vi "Create.vi"(6 "exchange name":string, 7 "instance name":string, 8 "error in (no error)":errorcluster, 11 "service name":string) -> (0 "error out":errorcluster, 3 "publisher":refnum<class "IcmMessagePublisher.lvclass">)   [LabVIEW 2017, in "IcmMessagePublisher.lvclass"]
doc: "Creates an NI InsightCM Publisher message bus session."
uses:
  <vilib>/addons/InsightCM/MessageBus/MessagePublisher/IcmMessagePublisher.lvclass
  <vilib>/addons/InsightCM/MessageBus/MessagePublisher/controls/MessagePublisherData.ctl
  C:/Program Files (x86)/National Instruments/LabVIEW 2017/vi.lib/addons/InsightCM/Binaries/LabviewMessageAdapter.dll
  Binaries/LabviewMessageAdapter.dll
  <vilib>/addons/InsightCM/MessageBus/MessagePublisher/IcmMessagePublisher.lvclass/IcmMessagePublisher.ctl
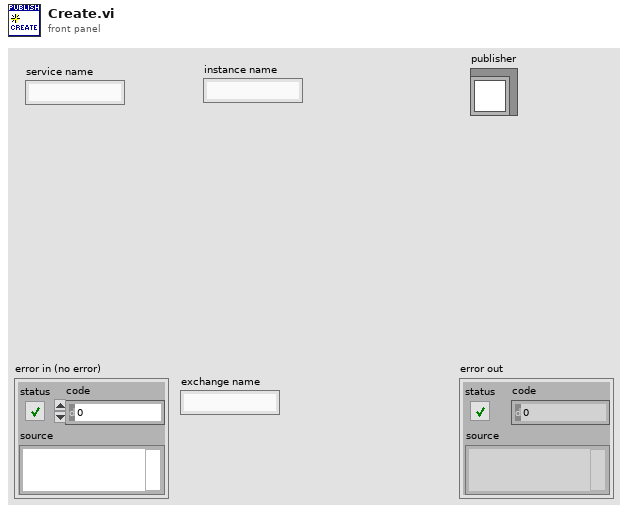
[diagram p1: front panel]
types:
  T1 = typedef "MessagePublisherData.ctl" = cluster{"Publisher":refnum<k24>}
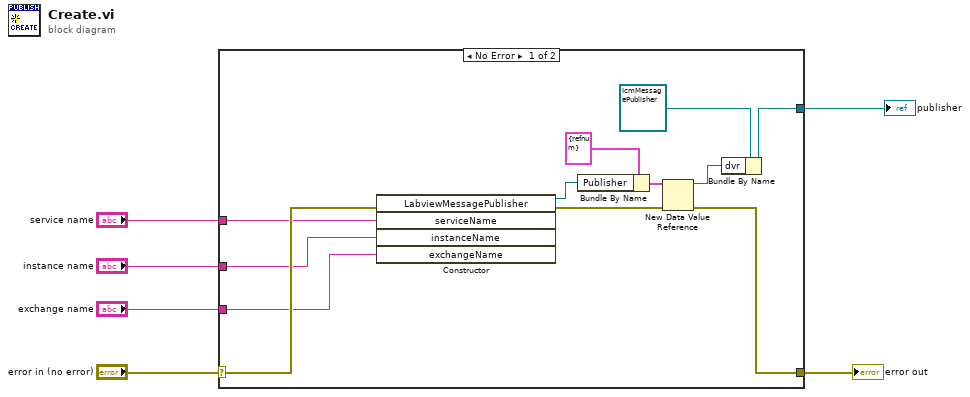
[diagram p0: block diagram]
diagram:
  n1 = case shown="No Error" "error in (no error)" {
    selector: "error in (no error)" -> [w11 w19]
    tunnel: [w10 w19] -> w5
    tunnel: [w12 _] -> w4
    tunnel: "service name" -> [w9 _]
    tunnel: "instance name" -> [w8 _]
    tunnel: "exchange name" -> [w7 _]
    frame No Error {
      n2 = constructor class="LabviewMessagePublisher"(error in=w11, "serviceName"=w9, "instanceName"=w8, "exchangeName"=w7) -> (reference out=w16:refnum<k24>, error out=w17:errorcluster)  [unwired: 2 in, 4 out]
      n3 = Bundle By Name(cluster=T1 {"Publisher"=refnum} ("Publisher"), "Publisher"=w16) -> (w18:T1)
      n4 = New Data Value Reference(data value=w18, error in=w17) -> (data value reference=w15:refnum<data-value>, error out=w10:errorcluster)
      n5 = Bundle By Name(cluster=refnum<class "IcmMessagePublisher.lvclass"> refnum ("IcmMessagePublisher in"), "dvr"=w15) -> (w12:refnum<class "IcmMessagePublisher.lvclass">)
    }
    frame Error {
    }
  }
  "error out" <- w5
  "publisher" <- w4
